vi "Get Lines.vi"(8 "error in (no error)":errorcluster, 11 "Polygon in":refnum<class "Polygon.lvclass">) -> (0 "error out":errorcluster, 2 "Lines":refnum<class "Line.lvclass">[](array[class]), 3 "Polygon out":refnum<class "Polygon.lvclass">)   [LabVIEW 2015, in "Polygon.lvclass"]
uses:
  Polygon.lvclass
  Line/Line.lvclass
  Polygon.lvclass/Polygon.ctl
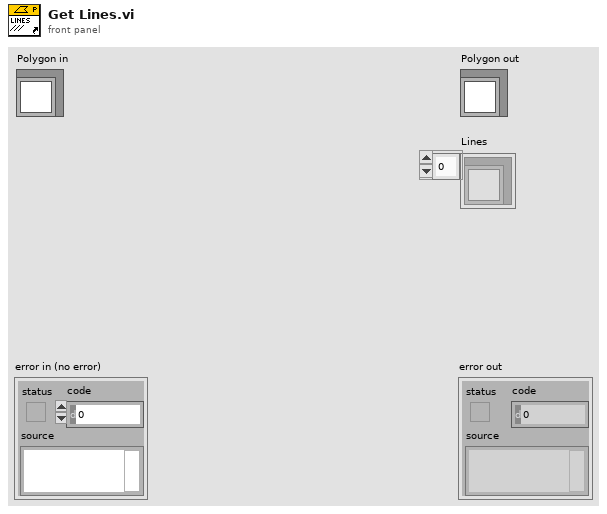
[diagram p1: front panel]
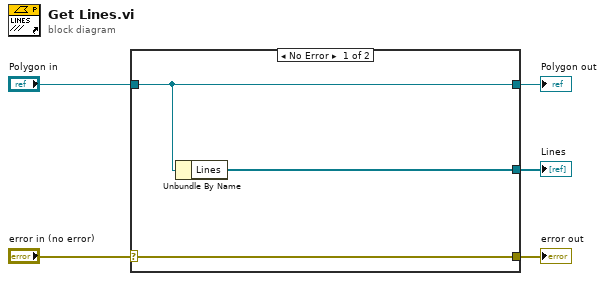
[diagram p0: block diagram]
diagram:
  n1 = case shown="No Error" "error in (no error)" {
    selector: "error in (no error)" -> [w8 w9]
    tunnel: [w8 w9] -> w4
    tunnel: [w7 w10] -> w2
    tunnel: "Polygon in" -> [w7 w10]
    tunnel: [w6 _] -> w1
    frame No Error {
      n2 = Unbundle By Name(w7) -> ("Lines"=w6:refnum<class "Line.lvclass">[])
    }
    frame Error {
    }
  }
  "error out" <- w4
  "Polygon out" <- w2
  "Lines" <- w1
